vi "acq.saveLight.EL.vi"(5 "vars":T2={"save"={"base_folder"={"Folder"=path "", "tif"=FALSE, "jpg"=FALSE}, "module"="", "#"=20, "sub#"=0, "save.op"=enum."Full", "same?"=FALSE, "Shift"=enum."Single", "jpg?"=FALSE, "flip"={"x"=FALSE, "y"=FALSE}}, "acq"={"# Acq"=100, "rotate"=FALSE}, "calib.manual"={"BG"={"Image"=[], "enabled?"=FALSE}, "FF"={"Image"=[], "enabled?"=FALSE}}}, 7 "path":T1, 8 "error in":errorcluster, 10 "EL":u16[][](array[numeric])) -> (0 "error out":errorcluster, 2 "EL":u16[][](array[numeric]))   [LabVIEW 2020]
uses:
  _controls/data.vars.ctl
  _controls/flip.ctl
  _controls/path.ctl
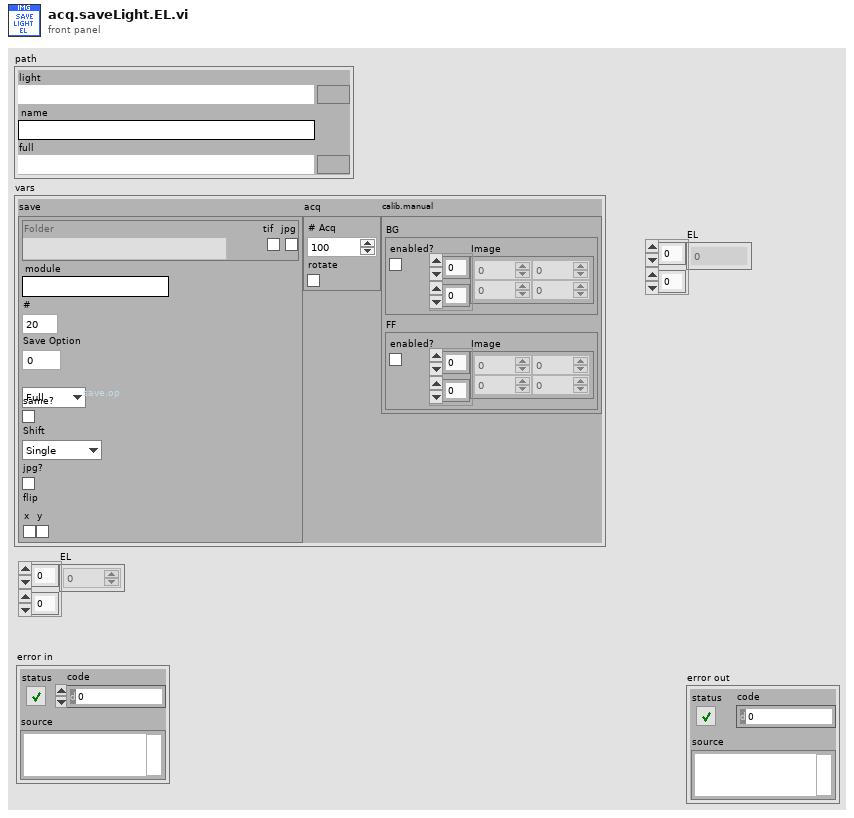
[diagram p1: front panel]
types:
  T1 = typedef "path.ctl" = cluster{"light":path, "name":string, "full":path}
  T2 = typedef "data.vars.ctl" = cluster{"save":cluster{"base_folder":cluster{"Folder":path, "tif":bool, "jpg":bool}, "module":string, "#":u32, "sub#":u8, "save.op":enum16{"Full", "Light"}, "same?":bool, "Shift":enum16{"Single", "Leapfrog"}, "jpg?":bool, "flip":T3}, "acq":cluster{"# Acq":u16, "rotate":bool}, "calib.manual":cluster{"BG":cluster{"Image":u16[][], "enabled?":bool}, "FF":cluster{"Image":u16[][], "enabled?":bool}}}
  T3 = typedef "flip.ctl" = cluster{"x":bool, "y":bool}
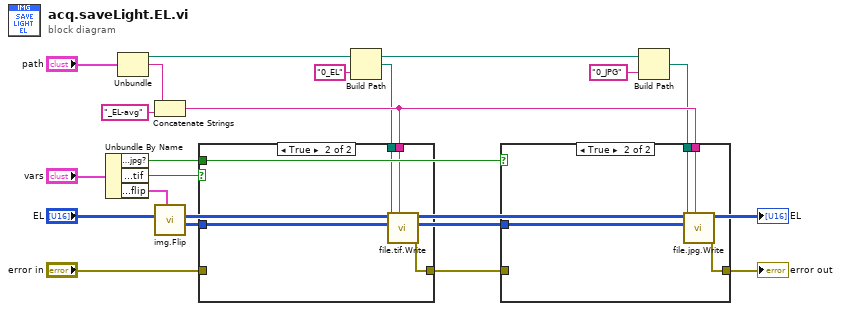
[diagram p0: block diagram]
diagram:
  n1 = Unbundle By Name("vars") -> ("save.jpg?"=w6:bool, "save.base_folder.tif"=w2:bool, "save.flip"=w1:T3)
  n2 = Unbundle("path") -> ("light"=w11:path, "name"=w3:string)  [unwired: 1 out]
  n3 = Concatenate Strings(w3, "_EL-avg" ("name or relative path")) -> (w15:string)
  n4 = call "img.Flip.vi"("flip"=w1, "image in"="EL") -> ("image out"=w9:u16[][])  [unwired: 9 in]
  n5 = Build Path(base path=w11, name or relative path="0_EL") -> (appended path=w10:path)
  n6 = case shown="True" w2 {
    tunnel: [w19 w23] -> w16
    tunnel: w9 -> [_ w22]
    tunnel: "error in" -> [w19 _]
    tunnel: w6 -> [_ _]
    tunnel: w15 -> [_ w21]
    tunnel: w10 -> [_ w20]
    frame False {
    }
    frame True {
      n7 = call "file.tif.Write.vi"("name"=w21, "u16 pixmap"=w22, "path"=w20) -> ("error out"=w23:errorcluster)  [unwired: 8 in]
    }
  }
  n8 = Build Path(base path=w11, name or relative path="0_JPG") -> (appended path=w13:path)
  n9 = case shown="True" w6 {
    tunnel: [w24 w28] -> w4
    tunnel: w9 -> [_ w27]
    tunnel: w13 -> [_ w26]
    tunnel: w16 -> [w24 _]
    tunnel: w15 -> [_ w25]
    frame False {
    }
    frame True {
      n10 = call "file.jpg.Write.vi"("name"=w25, "u16 pixmap"=w27, "path"=w26) -> ("error out"=w28:errorcluster)  [unwired: 8 in]
    }
  }
  "error out" <- w4
  "EL" <- "EL"
